vi "FMPA Retrieve Scan Data (single process).vi"(0 "System no.":i32=1 min=1 max=4 step=1, 2 "Process":string, 4 "Graph data?":bool, 5 "error in":errorcluster) -> (11 "Duration (msec)":u32, 14 "Max_Pos_(scan)":dbl=56.5106697, 16 "Max_Pos_(step)":dbl=75.2889633, 17 "Imax (V)":dbl=0.0006711610734750763 format="%.2e", 18 "Data":dbl[][](array[numeric]), 19 "error out":errorcluster)   [LabVIEW 2023]
uses:
  <vilib>/Native 3D Graph/xcontrol/3DPC_SurfacePlot.xctl
  <vilib>/Native 3D Graph/classes/Line/Line.lvclass
panel:
  out "Waveform Graph 3":dbl[](graph)
  out "Waveform Graph 2":dbl[](graph)
  out "Waveform Graph":dbl[](graph)
  out "max index(es)":i32
  out "max value":dbl
  out "size(s)":i32[](array[numeric])
  out "3D Line Graph":refnum<class "Base Datatype.lvclass">[](xcontrol)
  out "Position at max info":string="1=5.65106697E+001 2=7.52889633E+001"
  out "Scan successful?":bool=TRUE
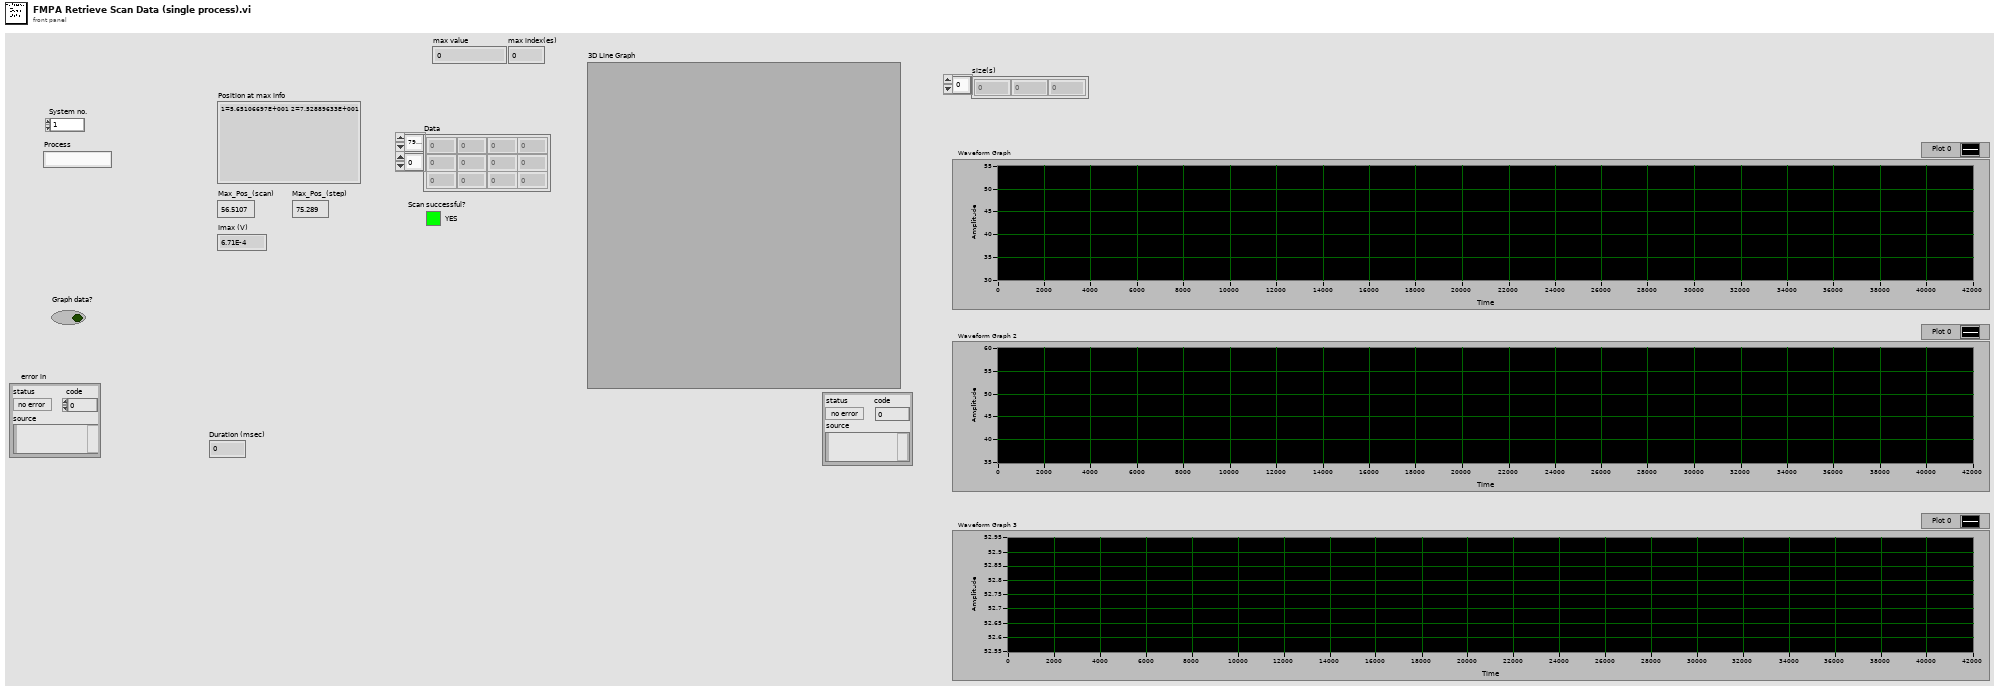
[diagram p1: front panel]
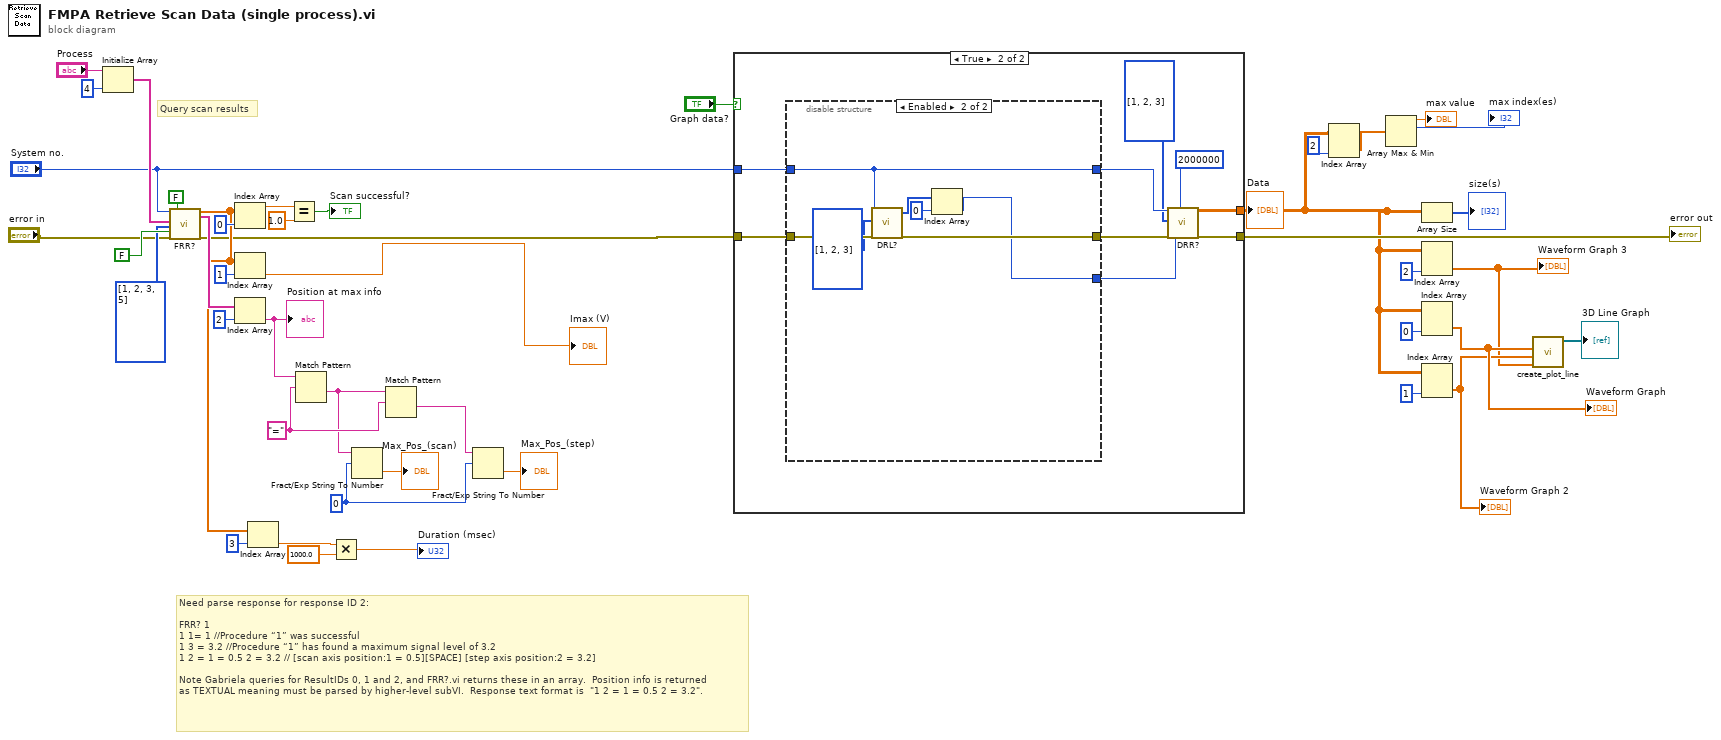
[diagram p0: block diagram]
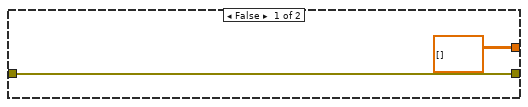
[diagram p2: hidden frame]
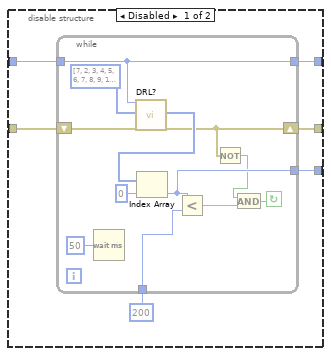
[diagram p3: hidden frame]
diagram:
  w31 = 0 ("offset")
  w32 = "=" ("regular expression")
  # "Query scan results"
  # "Need parse response for response ID 2:\n\nFRR? 1\n1 1= 1 //Procedure “1” was successful\n1 3 = 3.2 //Procedure “1” has found a maximum signal level of 3.2\n1 2 = 1 = 0.5 2 = 3.2 // [scan axis position:1 = 0.5][SPACE] [step axis position:2 = 3.2]\n\nNote Gabriela queries for ResultIDs 0, 1 and 2, and FRR?.vi returns these in an array.  Position info is returned \nas TEXTUAL meaning must be parsed by higher-level subVI.  Response text format is  \"1 2 = 1 = 0.5 2 = 3.2\"."
  n1 = Initialize Array("Process", 4 ("dimension size")) -> (w41:string[])
  n2 = call "FRR?.vi"("System no."="System no.", "Routinename"=w41, "ResultID"=i32[] [1, 2, 3, 5], "Query all?"=FALSE, "error in"="error in", "Use FRH?"=FALSE) -> ("Value (num.)"=w24:dbl[], "Value (string)"=w34:string[], "error out"=w11:errorcluster)  [unwired: 11 out]
  n3 = Index Array(array=w24, index=0) -> (element=w38:dbl)
  n4 = Index Array(array=w24, index=1) -> (element=→"Imax (V)":dbl)
  n5 = Index Array(array=w34, index=2) -> (element=w33:string)
  "Position at max info" <- w33
  n6 = Index Array(array=w24, index=3) -> (element=w23:dbl)
  n7 = Equal?(x=w38, y=1.0) -> (x = y?=→"Scan successful?":bool)
  n8 = Match Pattern(string=w33, regular expression=w32) -> (after substring=w28:string)  [unwired: 1 in, 3 out]
  n9 = Multiply(x=w23, y=1000.0) -> (x*y=→"Duration (msec)":dbl)
  n10 = Fract/Exp String To Number(string=w28, offset=w31) -> (number=→"Max_Pos_(scan)":dbl)  [unwired: 2 in, 1 out]
  n11 = Match Pattern(string=w28, regular expression=w32) -> (after substring=w27:string)  [unwired: 1 in, 3 out]
  n12 = Fract/Exp String To Number(string=w27, offset=w31) -> (number=→"Max_Pos_(step)":dbl)  [unwired: 2 in, 1 out]
  n13 = case shown="True" "Graph data?" {
    tunnel: "System no." -> [_ w53]
    tunnel: w11 -> [w46 w52]
    tunnel: [w46 w55] -> w12
    tunnel: [dbl[][] [] ("Data") w54] -> w8
    frame False {
    }
    frame True {
      n14 = disable-structure shown="Enabled" {
        disable-tunnel: w53 -> [w61 w74]
        disable-tunnel: w52 -> [w60 w80]
        disable-tunnel: [w59 w78] -> w51
        disable-tunnel: [w58 w74] -> w50
        disable-tunnel: [w56 w75] -> w48
        frame Disabled {
          n15 = while {
            tunnel: w61 -> [w71]
            shift-right: [w65] -> w59
            shift-left: w60 -> [w72]
            tunnel: [w71] -> w58
            tunnel: 200 ("N") -> [w68]
            tunnel: [w67] -> w56
            stop <- w64 continue-if-true
            n16 = Wait (ms)(milliseconds to wait=u32 50) -> ()  [unwired: 1 out]
            n17 = call "DRL?.vi"("System no."=w71, "Rec. table to query"=i32[] [7, 2, 3, 4, 5, 6, 7, 8, 9, 10, 11, 12], "error in"=w72) -> ("No. of rec. values"=w70:i32[], "error out"=w65:errorcluster)  [unwired: 1 in, 14 out]
            n18 = Index Array(array=w70, index=0) -> (element=w67:i32)
            n19 = Less?(x=w67, y=w68) -> (x < y?=w63:bool)
            n20 = Not(x=w65) -> (.not. x?=w62:bool)
            n21 = And(x=w62, y=w63) -> (x .and. y?=w64:bool)
          }
        }
        frame Enabled {
          n22 = call "DRL?.vi"("System no."=w74, "Rec. table to query"=i32[] [1, 2, 3], "error in"=w80) -> ("No. of rec. values"=w77:i32[], "error out"=w78:errorcluster)  [unwired: 15 in]
          n23 = Index Array(array=w77, index=0) -> (element=w75:i32)
        }
      }
      n24 = call "DRR?.vi"("System no."=w50, "Rec. table IDs"=i32[] [1, 2, 3], "error in"=w51, "N"=w48, "Nmax"=2000000) -> ("Data"=w54:dbl[][], "error out"=w55:errorcluster)  [unwired: 3 in, 10 out]
    }
  }
  "Data" <- w8
  "error out" <- w12
  n25 = Index Array(array=w8, index (col)=2 ("index (row)")) -> (element=w7:dbl[])  [unwired: 1 in]
  n26 = Array Max & Min(array=w7) -> (max value=→"max value":dbl, max index (indices)=→"max index(es)":i32)  [unwired: 2 out]
  n27 = Array Size(array=w8) -> (size(s)=→"size(s)":i32[])
  n28 = Index Array(array=w8, index (col)=2 ("index")) -> (element=w1:dbl[])  [unwired: 1 in]
  "Waveform Graph 3" <- w1
  n29 = Index Array(array=w8, index (col)=0 ("index")) -> (element=w3:dbl[])  [unwired: 1 in]
  "Waveform Graph" <- w3
  n30 = Index Array(array=w8, index (col)=1 ("index")) -> (element=w2:dbl[])  [unwired: 1 in]
  "Waveform Graph 2" <- w2
  n31 = call <vilib>:"create_plot_line.vi"("z vector"=w1, "y vector"=w2, "x vector"=w3) -> ("plots out"=→"3D Line Graph":refnum<class "Base Datatype.lvclass">[])  [unwired: 2 in, 6 out]
